vi "PC_DDPG to DDPM DAQ1 to DAQ2.vi"() -> ()   [LabVIEW 2021]
uses:
  Common/Typedefs/Execution Options - Measure.ctl
  Dynamic Digital Pattern Measurement/Typedefs/Timing & Trigger Settings.ctl
  Dynamic Digital Pattern Measurement/Typedefs/Timing Settings.ctl
  Dynamic Digital Pattern Measurement/Typedefs/Trigger Settings.ctl
  Synchronization/Typedefs/Routing Path.ctl
  Synchronization/Typedefs/Routing Signal.ctl
  Dynamic Digital Pattern Measurement/DAQ_Dynamic Digital Pattern Measurement.lvlib
  Synchronization/DAQ_Synchronization.lvlib
  Dynamic Digital Pattern Generation/DAQ_Dynamic Digital Pattern Generation.lvlib
panel:
  out "Port Digital Data Out":u32[](array[numeric])
  out "Port Digital Data In":u32[](array[numeric])
  out "Measured Digital Patterns":digitalwaveform(graph)={"t0"=timestamp(3805344626.9446526 s since 1904-01-01), "dt"=9.999999999999999e-05, "Y"={"transitions"=[], "data"=array65534x16[1048544 elements]}, "attributes"=variant("NI_ChannelName"=variant(string "Dev2/port0/line0..."), "NI_LineNames"=variant(string "Dev2/port0/line0,Dev2/port0/line1,Dev2/port0/line2,Dev2/port0/line3,Dev2/port0/line4,Dev2/port0/line5,Dev2/port0/line6,Dev2/port0/line7,Dev2/port0/line8,Dev2/port0/line9,Dev2/port0/line10,Dev2/port0/line11,Dev2/port0/line12,Dev2/port0/line13,Dev2/port0/line14,Dev2/port0/line15"))}
  out "error out":errorcluster
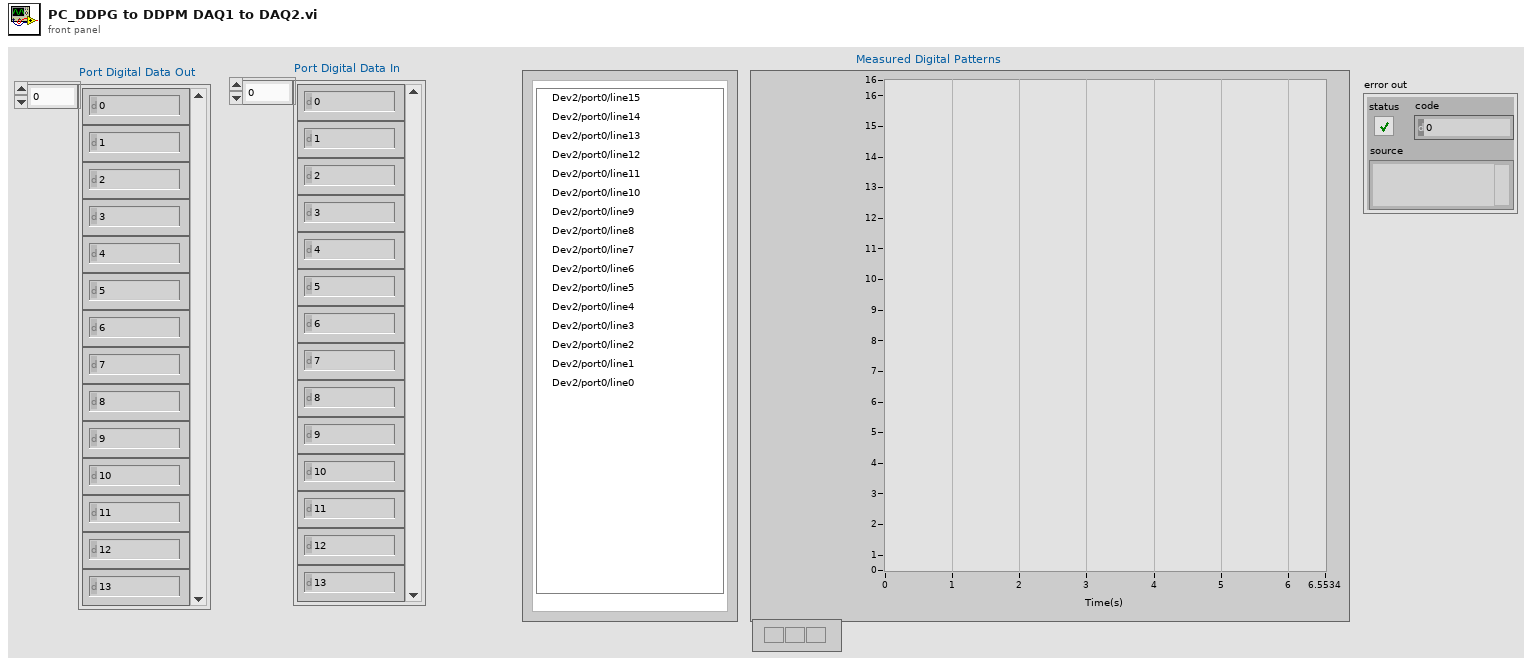
[diagram p1: front panel]
types:
  T1 = typedef "DAQ_Synchronization.lvlib/Routing Path.ctl" = cluster{"Signal":T2, "Output Terminal":tag}
  T2 = typedef "DAQ_Synchronization.lvlib/Routing Signal.ctl" = enum16{"Sample Clock", "Start Trigger"}
  T3 = typedef "DAQ_Dynamic Digital Pattern Measurement.lvlib/Timing & Trigger Settings.ctl" = cluster{"Timing Settings":T4, "Trigger Settings":T5}
  T4 = typedef "DAQ_Dynamic Digital Pattern Measurement.lvlib/Timing Settings.ctl" = cluster{"Sample Clock Source":tag, "Sample Rate (Hz)":dbl, "Number of Samples":i32, "Active Edge":i32}
  T5 = typedef "DAQ_Dynamic Digital Pattern Measurement.lvlib/Trigger Settings.ctl" = cluster{"Trigger Type":enum16{"No Trigger", "Digital Start"}, "Digital Start Trigger Source":tag, "Digital Start Trigger Edge":i32}
  T6 = typedef "Execution Options - Measure.ctl" = enum16{"Configure & Measure", "Configure only", "Measure only"}
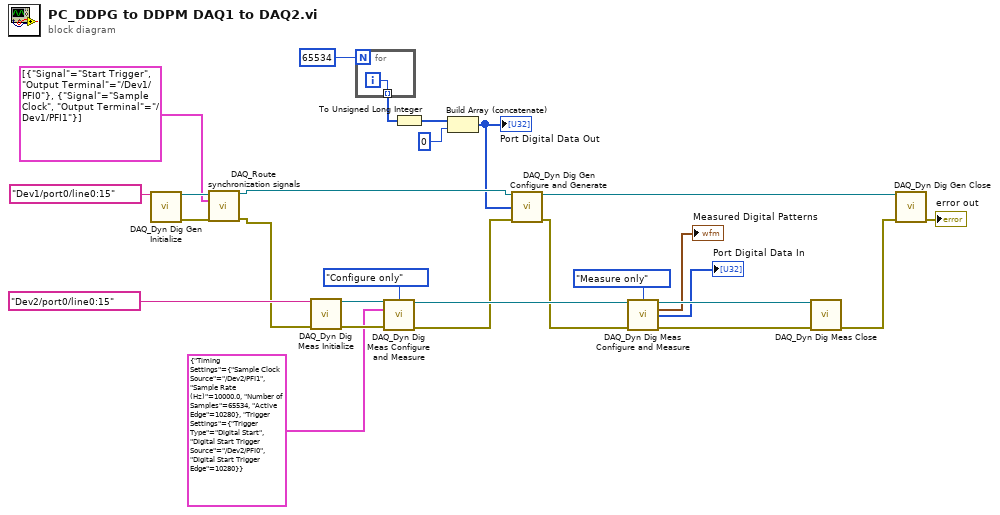
[diagram p0: block diagram]
diagram:
  n1 = call "DAQ_Dyn Dig Gen Initialize.vi"("Physical Channels"=tag "Dev1/port0/line0:15") -> ("DAQmx Task Out"=w11:refnum<k21>, "error out"=w10:errorcluster)  [unwired: 13 in]
  n2 = call "DAQ_Route synchronization signals.vi"("DAQmx Task In"=w11, "Routing paths"=T1[] [{"Signal"=enum."Start Trigger", "Output Terminal"="/Dev1/PFI0"}, {"Signal"=enum."Sample Clock", "Output Terminal"="/Dev1/PFI1"}], "error in"=w10) -> ("DAQmx Task Out"=w8:refnum<k21>, "error out"=w9:errorcluster)  [unwired: 11 in]
  n3 = call "DAQ_Dyn Dig Meas Initialize.vi"("Physical Channels"=tag "Dev2/port0/line0:15", "error in"=w9) -> ("DAQmx Task Out"=w25:refnum<k21>, "error out"=w23:errorcluster)  [unwired: 12 in]
  n4 = for {
    N: 65534 -> [_]
    tunnel: [w28] -> w4 mode=indexing
    i -> [w28]
  }
  n5 = call "DAQ_Dyn Dig Meas Configure and Measure.vi"("DAQmx Task In"=w25, "Execution Option"=Execution_Options_-_Measure."Configure only", "Timing and Trigger Settings"=T3 {"Timing Settings"={"Sample Clock Source"="/Dev2/PFI1", "Sample Rate (Hz)"=10000.0, "Number of Samples"=65534, "Active Edge"=10280}, "Trigger Settings"={"Trigger Type"=enum."Digital Start", "Digital Start Trigger Source"="/Dev2/PFI0", "Digital Start Trigger Edge"=10280}}, "error in"=w23) -> ("DAQmx Task Out"=w24:refnum<k21>, "error out"=w22:errorcluster)  [unwired: 7 in, 3 out]
  n6 = To Unsigned Long Integer(number=w4) -> (unsigned 32bit integer=w3:u32[])
  n7 = Build Array (concatenate)(w3, u32 0 ("new element/subarray")) -> (w1:u32[])
  "Port Digital Data Out" <- w1
  n8 = call "DAQ_Dyn Dig Gen Configure and Generate.vi"("DAQmx Task In"=w8, "Port Digital Data"=w1, "error in"=w22) -> ("DAQmx Task Out"=w26:refnum<k21>, "error out"=w21:errorcluster)  [unwired: 10 in, 1 out]
  n9 = call "DAQ_Dyn Dig Meas Configure and Measure.vi"("DAQmx Task In"=w24, "Execution Option"=Execution_Options_-_Measure."Measure only", "error in"=w21) -> ("DAQmx Task Out"=w19:refnum<k21>, "Measured Digital Patterns"=→"Measured Digital Patterns":digitalwaveform, "Port Digital Data"=→"Port Digital Data In":u32[], "error out"=w20:errorcluster)  [unwired: 8 in, 1 out]
  n10 = call "DAQ_Dyn Dig Meas Close.vi"("DAQmx Task In"=w19, "error in"=w20) -> ("error out"=w18:errorcluster)  [unwired: 13 in]
  n11 = call "DAQ_Dyn Dig Gen Close.vi"("DAQmx Task In"=w26, "error in"=w18) -> ("error out"=→"error out":errorcluster)  [unwired: 13 in]
